vi "menuActivate.vi"(8 "error in (no error)":errorcluster, 10 "flatMenu[] in":T1, 11 "Parameters in":refnum<class "Parameters.lvclass">) -> (0 "error out":errorcluster, 2 "flatMenu[] out":T1, 3 "Parameter out":refnum<class "Parameters.lvclass">)   [LabVIEW 2013, in "Parameters.lvclass"]
doc: "Takes the relevent data of the xceDataNode, and produces an array which represents the menu options in the tree control."
uses:
  Parameters.lvclass
  xCE/_shared/flatMenu.ctl
  xCE/xceDataNode/xceDataNode.lvclass
  xCE/xceNode/xceNode.lvclass
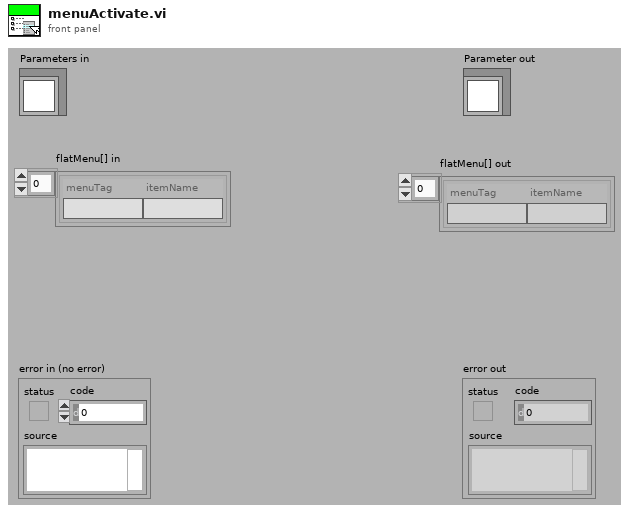
[diagram p1: front panel]
types:
  T1 = typedef "flatMenu.ctl" = cluster{"menuTag":string, "itemName":string}[]
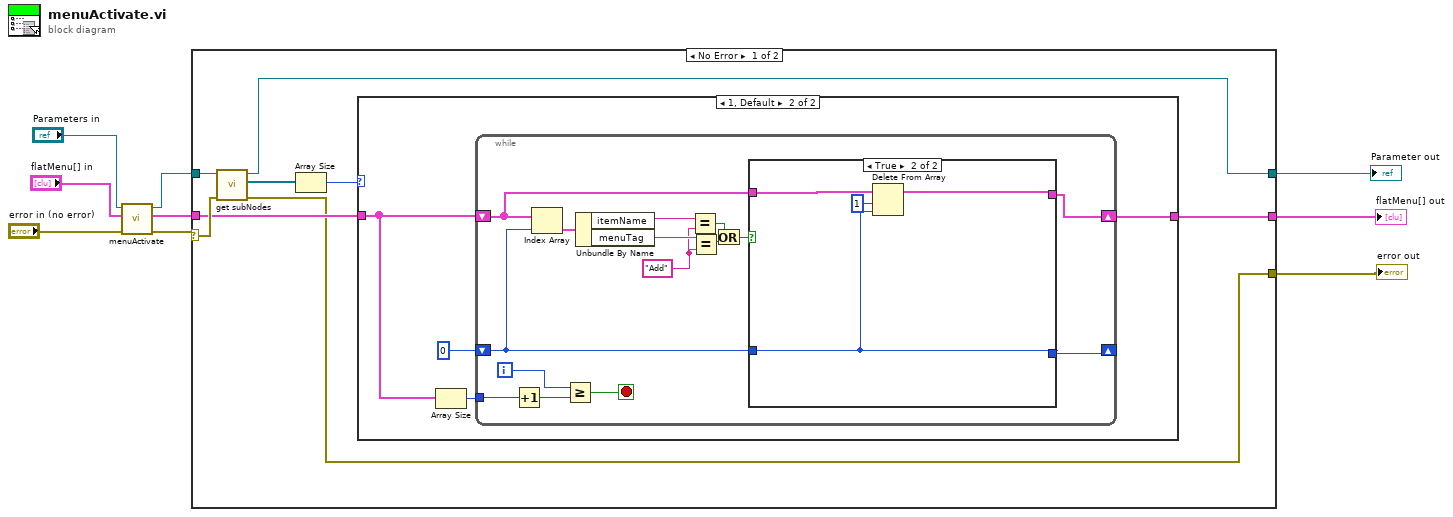
[diagram p0: block diagram]
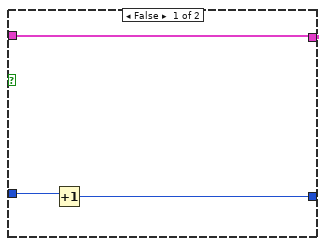
[diagram p3: hidden frame]
diagram:
  n1 = call-parent "menuActivate.vi"("error in (no error)"="error in (no error)", "flatMenu[] in"="flatMenu[] in", "xceDataNode in"="Parameters in") -> ("error out"=w6:errorcluster, "flatMenu[] out"=w5:T1, "xceDataNode out"=w4:refnum<class "Parameters.lvclass">)  [unwired: 6 in]
  n2 = case shown="No Error" w6 {
    selector: w6 -> [w16 w44]
    tunnel: w5 -> [w13 w45]
    tunnel: w4 -> [w17 w46]
    tunnel: [w12 w46] -> w3
    tunnel: [w11 w45] -> w2
    tunnel: [w10 w44] -> w1
    frame No Error {
      n3 = call "get subNodes.vi"("error in (no error)"=w16, "xceNode in"=w17) -> ("error out"=w10:errorcluster, "subNodes[]*"=w15:refnum<data-value>[], "xceNode out"=w12:refnum<class "Parameters.lvclass">)  [unwired: 7 in]
      n4 = Array Size(array=w15) -> (size(s)=w14:i32)
      n5 = case shown="1, Default" w14 {
        tunnel: w13 -> [w18 w22]
        tunnel: [w18 w19] -> w11
        frame 0 {
        }
        frame 1, Default {
          n6 = Array Size(array=w22) -> (size(s)=w21:i32)
          n7 = while {
            shift-right: [w31] -> w19
            shift-left: w22 -> [w32]
            shift-right: [w29] -> _
            shift-left: 0 -> [w30]
            tunnel: w21 -> [w28]
            i -> [w34]
            stop <- w33 stop-if-true
            w26 = "Add" ("y")
            n8 = Increment(x=w28) -> ()  [unwired: 1 out]
            n9 = Index Array(array=w32, index=w30) -> (element=w36:cluster{"menuTag":string, "itemName":string})
            n10 = Greater Or Equal?(x=w34, y=w28) -> (x >= y?=w33:bool)
            n11 = Unbundle By Name(w36) -> ("itemName"=w27:string, "menuTag"=w35:string)
            n12 = Equal?(x=w27, y=w26) -> (x = y?=w24:bool)
            n13 = Equal?(x=w35, y=w26) -> (x = y?=w23:bool)
            n14 = Or(x=w24, y=w23) -> (x .or. y?=w25:bool)
            n15 = case shown="True" w25 {
              tunnel: w32 -> [w37 w43]
              tunnel: [w37 w42] -> w31
              tunnel: w30 -> [w39 w41]
              tunnel: [w38 w41] -> w29
              frame False {
                n16 = Increment(x=w39) -> (x+1=w38:i32)
              }
              frame True {
                n17 = Delete From Array(array=w43, length=1, index=w41) -> (array with subset deleted=w42:T1)  [unwired: 1 out]
              }
            }
          }
        }
      }
    }
    frame Error {
    }
  }
  "error out" <- w1
  "Parameter out" <- w3
  "flatMenu[] out" <- w2
